vi "Get_Parent_Applies.vi"(8 "error in (no error)":errorcluster, 11 "AB_Source_Library in":refnum<class "AB_Source_Library.lvclass">) -> (0 "error out":errorcluster, 2 "parentApplies":T1, 3 "AB_Source_Library out":refnum<class "AB_Source_Library.lvclass">)   [LabVIEW 2020, in "AB_Source_Library.lvclass"]
uses:
  <vilib>/AppBuilder/AB_Classes/Source/Library/AB_Source_Library.lvclass
  <vilib>/AppBuilder/AB_Parent_Applies.ctl
  e:/builds/penguin/labview/branches/2020/dev/dist/vi.lib/AppBuilder/AB_Classes/Source/AB_Source.lvclass
  <vilib>/AppBuilder/AB_Source_Inclusion.ctl
  <vilib>/AppBuilder/AB_Classes/Source/Library/AB_Source_Library.lvclass/AB_Source_Library.ctl
  <vilib>/AppBuilder/AB_Classes/Source/AB_Source.lvclass
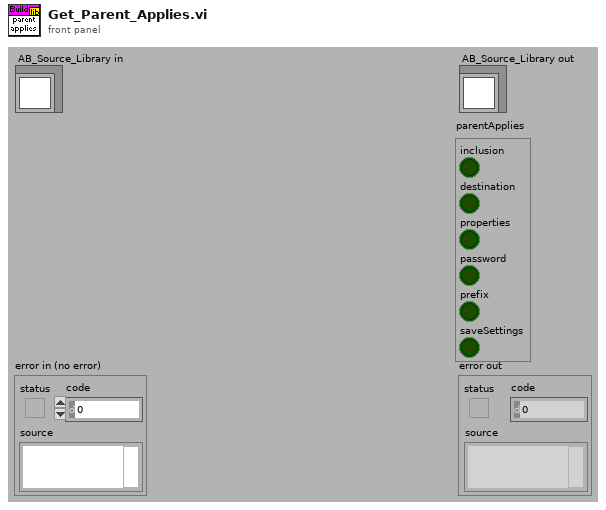
[diagram p1: front panel]
types:
  T1 = typedef "AB_Parent_Applies.ctl" = cluster{"inclusion":bool, "destination":bool, "properties":bool, "password":bool, "prefix":bool, "saveSettings":bool}
  T2 = typedef "AB_Source_Inclusion.ctl" = enum16{"IncludeIfReferenced", "Include", "Exclude", "TopLevel"}
  T3 = typedef "AB_Source.ctl" = cluster{"path":path, "itemID":string, "parentIndex":i32, "sourceInclusion":T2, "destinationIndex":i32, "properties":T4[], "newName":string, "lvfile":bool, "valid":bool, "eng_inBuild":bool, "eng_isNonVILink":bool, "Amalgamation":bool, "Amalgamation Piece":bool, "eng_delimitedName":string, "preventRename":bool}
  T4 = typedef "AB_Source_Properties.ctl" = cluster{"sourcePropertyType":T5, "value":variant}
  T5 = typedef "AB_Source_Property_Type.ctl" = enum16{"Remove block diagram", "Remove front panel", "Password", "Window has title bar", "Show menu bar", "Show vertical scroll bar", "Show horizontal scroll bar", "Show toolbar", "Show Abort button", "Show fp when called", "Window behavior", "Allow user to close window", "Window run-time position", "Run when opened", "Allow debugging", "Auto error handling", "Generate guard code", "Use stack variables", "Expression folding", "Integer only", "Inline subVI"}
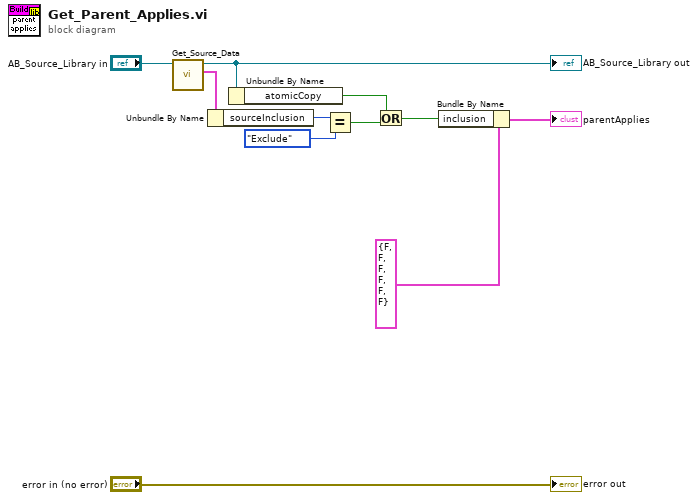
[diagram p0: block diagram]
diagram:
  n1 = call <vilib>:"Get_Source_Data.vi"("Class in"="AB_Source_Library in") -> ("data"=w4:T3, "Class out"=w5:refnum<class "AB_Source_Library.lvclass">)  [unwired: 8 in, 1 out]
  "AB_Source_Library out" <- w5
  n2 = Unbundle By Name(w4) -> ("sourceInclusion"=w3:T2)
  n3 = Unbundle By Name(w5) -> ("atomicCopy"=w8:bool)
  n4 = Equal?(x=w3, y=AB_Source_Inclusion."Exclude") -> (x = y?=w2:bool)
  n5 = Or(x=w8, y=w2) -> (x .or. y?=w7:bool)
  n6 = Bundle By Name(cluster=T1 {"inclusion"=FALSE, "destination"=FALSE, "properties"=FALSE, "password"=FALSE, "prefix"=FALSE, "saveSettings"=FALSE} ("parentApplies"), "inclusion"=w7) -> (→"parentApplies":T1)
  "error out" <- "error in (no error)"
